vi "Read Axi.In.vi"(8 "error in (no error)":errorcluster, 11 "Ethernet MAC - Custom in":refnum<class "Ethernet MAC - Custom.lvclass">) -> (0 "error out":errorcluster, 2 "Axi.In":T1, 3 "Ethernet MAC - Custom out":refnum<class "Ethernet MAC - Custom.lvclass">)   [LabVIEW 2020, in "Ethernet MAC - Custom.lvclass"]
uses:
  Ethernet MAC - Custom.lvclass
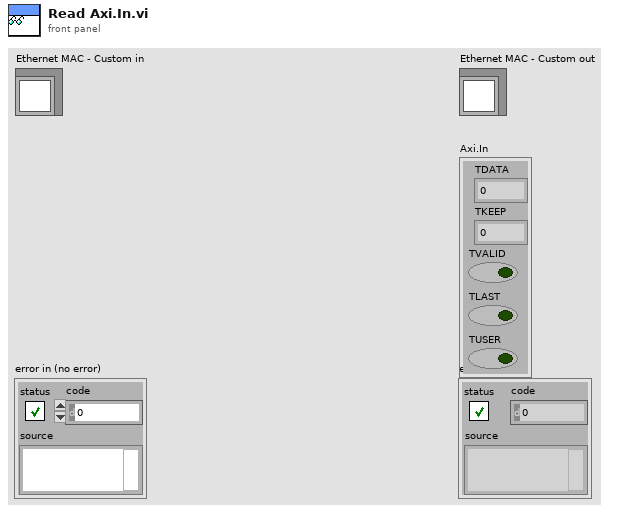
[diagram p1: front panel]
types:
  T1 = cluster{"TDATA":u64, "TKEEP":u8, "TVALID":bool, "TLAST":bool, "TUSER":bool}
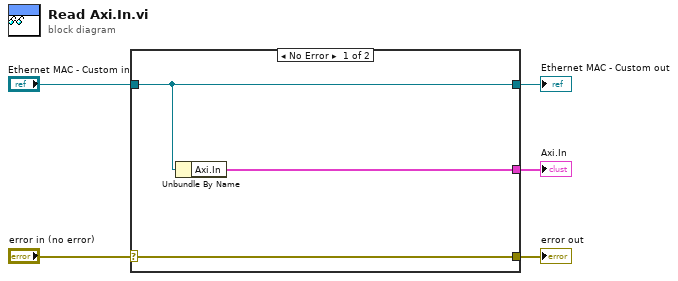
[diagram p0: block diagram]
diagram:
  n1 = case shown="No Error" "error in (no error)" {
    selector: "error in (no error)" -> [w8 w9]
    tunnel: [w8 w9] -> w4
    tunnel: [w7 w10] -> w2
    tunnel: "Ethernet MAC - Custom in" -> [w7 w10]
    tunnel: [w6 _] -> w1
    frame No Error {
      n2 = Unbundle By Name(w7) -> ("Axi.In"=w6:T1)
    }
    frame Error {
    }
  }
  "error out" <- w4
  "Ethernet MAC - Custom out" <- w2
  "Axi.In" <- w1
